vi "Check Channel Status.vi"(0 "fpga interface in":refnum<k20>, 5 "serial output channels":string[](array[string]), 11 "error in (no error)":errorcluster) -> (4 "fpga interface out":refnum<k20>, 6 "packet timing errors":bool[](array[boolean]), 8 "number of generated packets":u64[](array[numeric]), 15 "error out":errorcluster)   [LabVIEW 2023, in "GettingStarted_Gen_148X_Host.lvlib"]
uses:
  GettingStarted_Gen_148X_Host.lvlib
  Types/148x_Gen_FPGA_Reference.ctl
  <vilib>/rvi/errors/niLvFpgaAdjustHostInterfaceError.vi
  <vilib>/rvi/interface/nirviReadWriteControl/nirviReadWriteControl.xnode
  <instrlib>/FlexRIO/Automotive Vision Utility/v1/Host/Automotive Vision Utility.lvlib
  NiFpgaLv.dll
  <vilib>/rvi/interface/Simulation/niFpgaSimulationCallBeginRW.vi
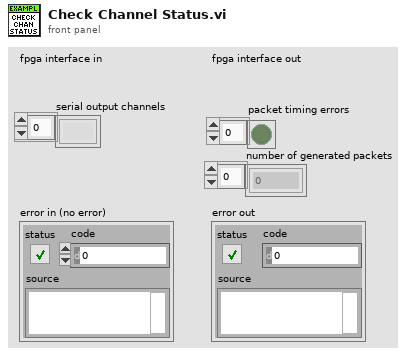
[diagram p1: front panel]
types:
  T1 = typedef "GettingStarted_Gen_148X_Host.lvlib/148x_Gen_FPGA_Reference.ctl" = refnum<k20>
  T2 = cluster{"num buffered llp packets":fxp<+,14,14>, "packet timing error (cycles)":u64, "packet timing error":bool, "ready to generate packet":bool, "dram status":cluster{"bytes written":u64, "bytes read":u64, "overflow":bool, "partition full":bool, "last byte flushed":bool}, "num buffered llp timestamps":u32, "generation done":bool, "num generated packets":u64}[]
  T3 = typedef "Automotive Vision Utility.lvlib/Serial Channel Type.ctl" = enum16{"Serial Input Channel", "Serial Output Channel", "Unknown Channel Type"}
  T4 = cluster{"num buffered llp packets":fxp<+,14,14>, "packet timing error (cycles)":u64, "packet timing error":bool, "ready to generate packet":bool, "dram status":cluster{"bytes written":u64, "bytes read":u64, "overflow":bool, "partition full":bool, "last byte flushed":bool}, "num buffered llp timestamps":u32, "generation done":bool, "num generated packets":u64}
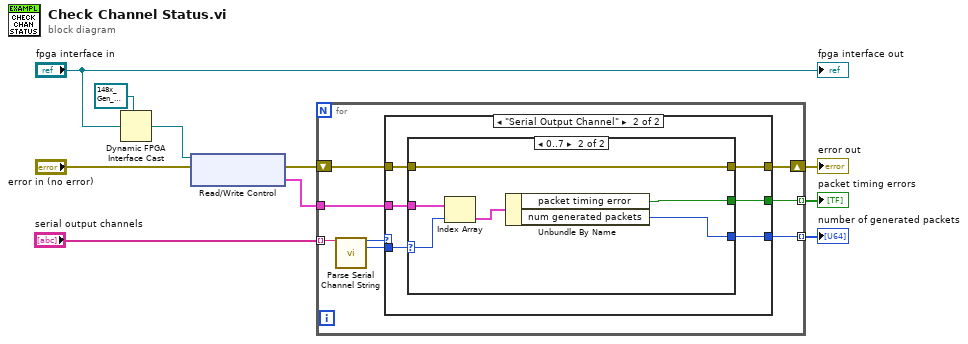
[diagram p0: block diagram]
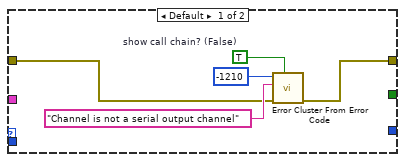
[diagram p2: hidden frame]
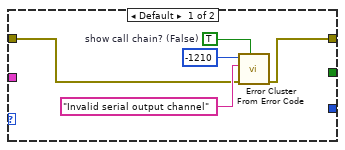
[diagram p3: hidden frame]
diagram:
  n1 = Dynamic FPGA Interface Cast(Session In=T1 refnum ("FPGA VI Reference Out"), Type="fpga interface in") -> (Session Out=w8:T1)
  n2 = xnode "Read/Write Control"("FPGA VI Reference In"=w8, "error in"="error in (no error)") -> ("error out"=w3:errorcluster, "channel status"=w6:T2)  [unwired: 1 out]
  n3 = for {
    tunnel: w6 -> [w18]
    tunnel: [w17] -> w2 mode=indexing
    tunnel: "serial output channels" -> [w16] mode=indexing
    shift-right: [w14] -> w4
    shift-left: w3 -> [w13]
    tunnel: [w11] -> w1 mode=indexing
    n4 = call <instrlib>:"Parse Serial Channel String.vi"("serial channel string"=w16) -> ("serial channel type"=w15:T3, "channel number"=w12:i32)  [unwired: 13 in]
    n5 = case shown="\"Serial Output Channel\"" w15 {
      tunnel: w18 -> [_ w28]
      tunnel: [_ w29] -> w17
      tunnel: [w20 w25] -> w14
      tunnel: w13 -> [w19 w26]
      tunnel: w12 -> [_ w27]
      tunnel: [_ w24] -> w11
      frame Default {
        w21 = TRUE  # show call chain? (False)
        n6 = call <vilib>:"Error Cluster From Error Code.vi"("show call chain? (False)"=w21, "error in (no error)"=w19, "error message (\"\")"="Channel is not a serial output channel" ("error message (\"\")"), "error code (0)"=-1210) -> ("error out"=w20:errorcluster)  [unwired: 5 in]
      }
      frame "Serial Output Channel" {
        n7 = case shown="0..7" w27 {
          selector: w27 -> [_ w37]
          tunnel: [_ w40] -> w29
          tunnel: w28 -> [_ w39]
          tunnel: w26 -> [w31 w36]
          tunnel: [w30 w36] -> w25
          tunnel: [_ w35] -> w24
          frame Default {
            w33 = TRUE  # show call chain? (False)
            n8 = call <vilib>:"Error Cluster From Error Code.vi"("show call chain? (False)"=w33, "error in (no error)"=w31, "error message (\"\")"="Invalid serial output channel" ("error message (\"\")"), "error code (0)"=-1210) -> ("error out"=w30:errorcluster)  [unwired: 5 in]
          }
          frame 0..7 {
            n9 = Index Array(array=w39, index=w37) -> (element=w38:T4)
            n10 = Unbundle By Name(w38) -> ("packet timing error"=w40:bool, "num generated packets"=w35:u64)
          }
        }
      }
    }
  }
  "error out" <- w4
  "packet timing errors" <- w2
  "number of generated packets" <- w1
  "fpga interface out" <- "fpga interface in"
